vi "SR830-Check-Port.vi"(8 "error in (no error)":errorcluster, 11 "SR830 in":refnum<vi>) -> (0 "error out":errorcluster, 2 "Boolean":bool, 3 "Sr830 out":refnum<vi>)   [LabVIEW 2016]
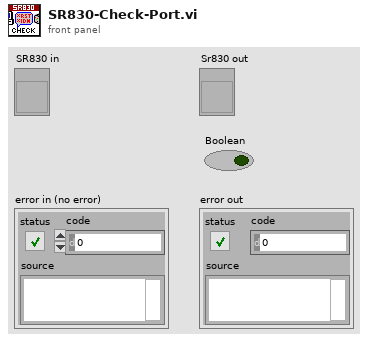
[diagram p1: front panel]
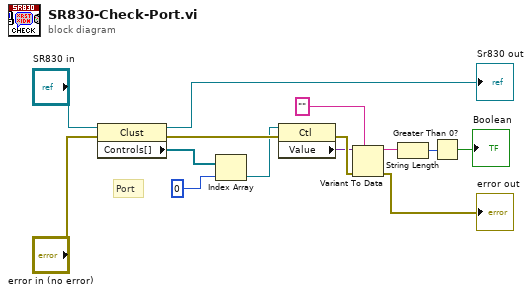
[diagram p0: block diagram]
diagram:
  # "Port"
  n1 = property class="Clust"(reference="SR830 in", error in="error in (no error)") -> (reference out=→"Sr830 out":refnum<vi>, error out=w6:errorcluster, "Controls[]"=w3:refnum<vi>[])
  n2 = Index Array(array=w3, index=0) -> (element=w5:refnum<vi>)
  n3 = property class="Ctl"(reference=w5, error in=w6) -> (error out=w9:errorcluster, "Value"=w8:variant)  [unwired: 1 out]
  n4 = Variant To Data(error in=w9, type="", Variant=w8) -> (data=w11:string, error out=→"error out":errorcluster)
  n5 = String Length(string=w11) -> (length=w12:i32)
  n6 = Greater Than 0?(x=w12) -> (x > 0?=→"Boolean":bool)
